vi "serialWrite.vi"(8 "error in (no error)":errorcluster, 10 "text":string, 11 "Python":T1) -> (0 "error out":errorcluster, 3 "Num loops":i32)   [LabVIEW 2021]
uses:
  PythonCtrl.ctl
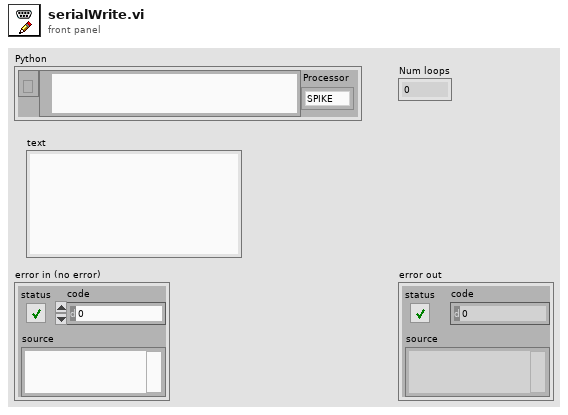
[diagram p1: front panel]
types:
  T1 = typedef "PythonCtrl.ctl" = cluster{"session":refnum<k35>, "PyPath":path, "Processor":enum16{"SPIKE", "Pi", "Pi_ssh"}}
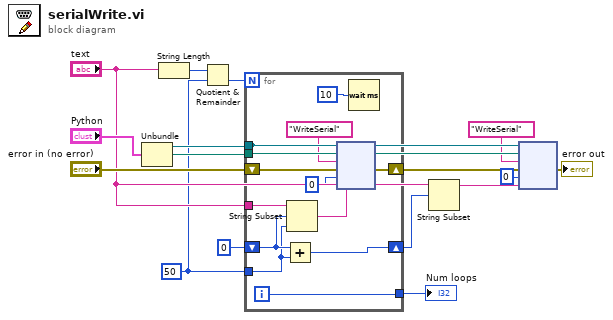
[diagram p0: block diagram]
diagram:
  w3 = 50 ("length (rest)")
  n1 = Unbundle("Python") -> ("session"=w15:refnum<k35>, "PyPath"=w16:path)  [unwired: 1 out]
  n2 = String Length(string="text") -> (length=w4:i32)
  n3 = Quotient & Remainder(x=w4, y=w3) -> (floor(x/y)=w2:i32)  [unwired: 1 out]
  n4 = for {
    N: w2 -> [_]
    tunnel: "text" -> [w29]
    shift-right: [w27] -> w1
    shift-left: 0 -> [w28]
    tunnel: w3 -> [w26]
    tunnel: [w24] -> w13
    shift-right: [w21] -> w10
    shift-left: "error in (no error)" -> [w20]
    tunnel: w15 -> [w18]
    tunnel: w16 -> [w17]
    i -> [w24]
    n5 = Add(x=w28, y=w26) -> (x+y=w27:i32)
    n6 = String Subset(string=w29, offset (0)=w28, length (rest)=w26) -> (substring=w22:string)
    n7 = node(w18, w17, "WriteSerial" ("function name"), w20, 0, w22) -> (w21:errorcluster)  [unwired: 2 in, 3 out]
    n8 = Wait (ms)(milliseconds to wait=u32 10) -> ()  [unwired: 1 out]
  }
  "Num loops" <- w13
  n9 = String Subset(string="text", offset (0)=w1) -> (substring=w11:string)  [unwired: 1 in]
  n10 = node(w15, w16, "WriteSerial" ("function name"), w10, 0, w11) -> (→"error out":errorcluster)  [unwired: 2 in, 3 out]
